vi "Home Stage.vi"(8 "error in (no error)":errorcluster, 11 "2-Axis Stage in":refnum<class "XY Stage Controller.lvclass">) -> (0 "error out":errorcluster, 3 "2-Axis Stage out":refnum<class "XY Stage Controller.lvclass">)   [LabVIEW 2022 SP3, in "XY Stage Controller.lvclass"]
uses:
  XY Stage Controller.lvclass
  XY Stage Controller.lvclass/XY Stage Controller.ctl
  XY Stage Process/XY Stage Process/XY Stage Process Messages/Home Stage Msg/Home Stage Msg.lvclass
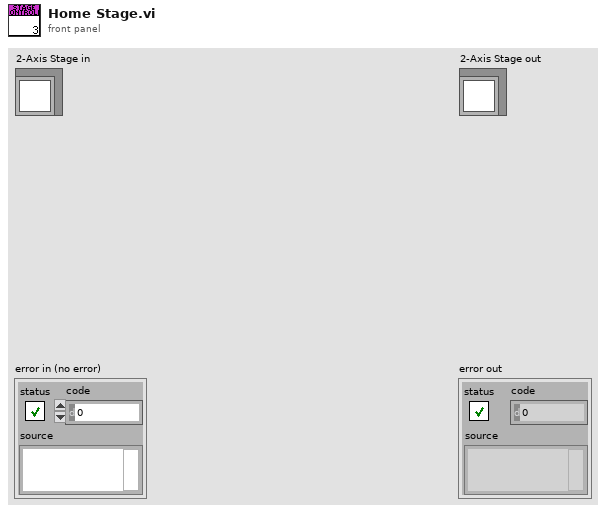
[diagram p1: front panel]
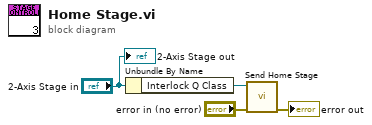
[diagram p0: block diagram]
diagram:
  n1 = Unbundle By Name("2-Axis Stage in") -> ("Interlock Q Class"=w3:refnum<class "Interlock Q Class.lvclass">)
  n2 = call "Send Home Stage.vi"("error in (no error)"="error in (no error)", "Interlock Q Class"=w3) -> ("error out"=→"error out":errorcluster)  [unwired: 8 in, 1 out]
  "2-Axis Stage out" <- "2-Axis Stage in"
